vi "Build UEGO Section from XML.vi"(4 "HW Settling Time":u32=250, 6 "Calibration Time":u32=1000, 7 "FPGA Item Name":string, 8 "error in (no error)":errorcluster, 9 "Card Position in":T1 {"Slot #" max=15}, 10 "Name in":string, 11 "Node Ptr in":u64) -> (0 "error out":errorcluster)   [LabVIEW 2014, in "SLSC configuration System Explorer.lvlib"]
uses:
  SLSC configuration System Explorer.lvlib
  Type Defs/Card Position.ctl
  Shared/SPI Utility/Slot #.ctl
  Shared/Constants.vi
  <vilib>/NI Veristand/Custom Device API/Set Item Property (U32).vi
  <vilib>/NI Veristand/Custom Device API/Set Item Property (String).vi
  <vilib>/NI Veristand/Custom Device API/Custom Device API.lvlib
  Shared/SLSC configuration Shared.lvlib
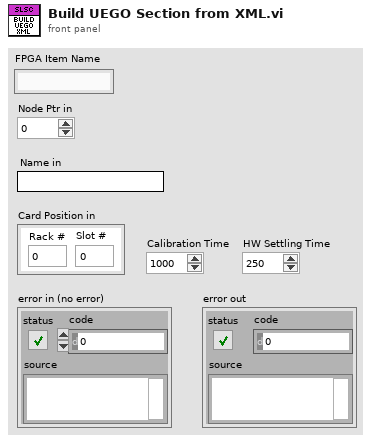
[diagram p1: front panel]
types:
  T1 = typedef "SLSC configuration Shared.lvlib/Card Position.ctl" = cluster{"Rack #":u8, "Slot #":T2}
  T2 = typedef "SLSC configuration Shared.lvlib/Slot #.ctl" = u8
  T3 = typedef "Custom Device API.lvlib/Custom Device Item Ref.ctl" = u64
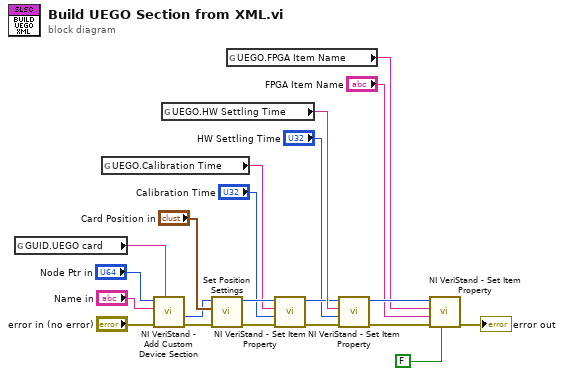
[diagram p0: block diagram]
diagram:
  n1 = global read "Constants.vi" "GUID.UEGO card"() -> (w16:string)
  n2 = global read "Constants.vi" "UEGO.Calibration Time"() -> (w11:string)
  n3 = call <vilib>:"NI VeriStand - Add Custom Device Section.vi"("GUID (Default Section)"=w16, "error in (no error)"="error in (no error)", "Section Name"="Name in", "Parent Ref in"="Node Ptr in") -> ("error out"=w15:errorcluster, "Section Ptr"=w14:T3)  [unwired: 4 in, 2 out]
  n4 = global read "Constants.vi" "UEGO.HW Settling Time"() -> (w10:string)
  n5 = call "Set Position Settings.vi"("error in (no error)"=w15, "Card Position"="Card Position in", "Item Ref in"=w14) -> ("error out"=w13:errorcluster, "Item Ref out"=w12:T3)  [unwired: 7 in]
  n6 = global read "Constants.vi" "UEGO.FPGA Item Name"() -> (w3:string)
  n7 = call-poly <vilib>:"NI VeriStand - Set Item Property.vi"("error in (no error)"=w13, "Value"="Calibration Time", "Property Name"=w11, "Item Ref in"=w12) -> ("error out"=w8:errorcluster, "Item Ref out"=w9:T3)  [unwired: 5 in, 1 out]
  n8 = call-poly <vilib>:"NI VeriStand - Set Item Property.vi"("error in (no error)"=w8, "Value"="HW Settling Time", "Property Name"=w10, "Item Ref in"=w9) -> ("error out"=w5:errorcluster, "Item Ref out"=w4:T3)  [unwired: 5 in, 1 out]
  n9 = call-poly <vilib>:"NI VeriStand - Set Item Property.vi"("Binary String (T)"=FALSE, "error in (no error)"=w5, "Value"="FPGA Item Name", "Property Name"=w3, "Item Ref in"=w4) -> ("error out"=→"error out":errorcluster)  [unwired: 4 in, 2 out]
